vi "write asci file.vi"(5 "Temp in":T1={"Vibr Chn Name"=[], "Analysis Chn Number"=0, "Index Vibration Waveform"={"t0"=timestamp(0 s since 1904-01-01), "dt"=1.0, "Y"=[]}, "Report Infomation"={"Test Name"="", "Tester"="", "Tempre Chart"=refnum, "Apli-Fre"=refnum, "Phase-Fre"=refnum, "Raw Data"=refnum}, "Vibr Apli - Fre"=[], "Vibr Phase - Fre"=[], "Error"={"status"=FALSE, "code"=0, "source"=""}, "Read Chan Name"="", "Test Info"={"Test Name"="", "Tester"=""}, "test data"=[{"t0"=timestamp(0 s since 1904-01-01), "dt"=1.0, "Y"=[]}, {"t0"=timestamp(0 s since 1904-01-01), "dt"=1.0, "Y"=[]}, {"t0"=timestamp(0 s since 1904-01-01), "dt"=1.0, "Y"=[]}, {"t0"=timestamp(0 s since 1904-01-01), "dt"=0.001, "Y"=[]}], "测试头文件"={"ch"=[], "测试环境"=""}, "CAl VAlUE"={"max_t"=[], "max_V"=[], "start_t"=[], "start_V"=[], "distance"=[], "unit"=""}}, 6 "unit":string[](array[string]), 7 "chanel name":string[](array[string]), 8 "error in (no error)":errorcluster, 9 "data":waveform(dbl)[](array[waveform]), 10 "格式":string, 11 "file (use dialog)":path) -> (0 "error out":errorcluster)   [LabVIEW 2011]
uses:
  Ctrls/ana data.ctl
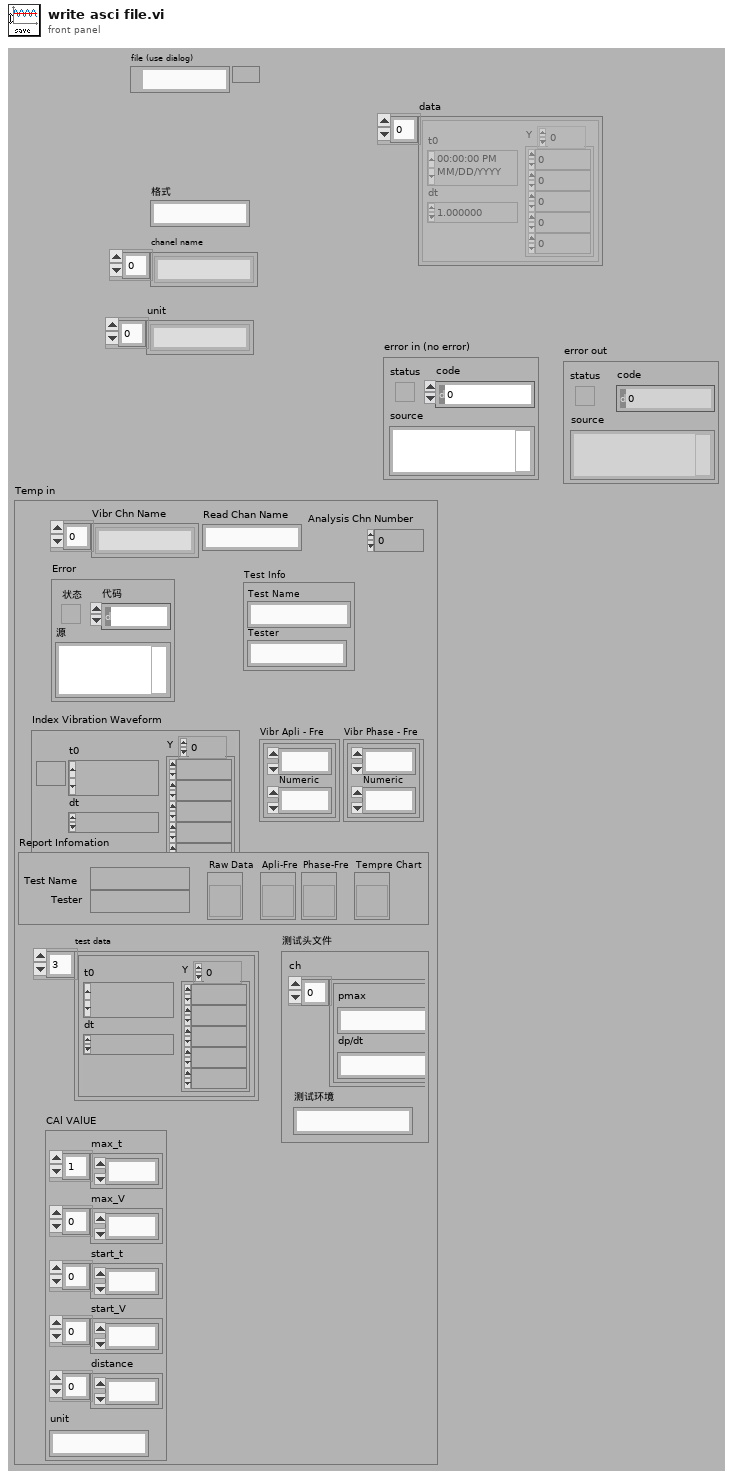
[diagram p1: front panel]
types:
  T1 = typedef "ana data.ctl" = cluster{"Vibr Chn Name":string[], "Analysis Chn Number":i32, "Index Vibration Waveform":waveform(dbl), "Report Infomation":cluster{"Test Name":string, "Tester":string, "Tempre Chart":refnum<vi>, "Apli-Fre":refnum<vi>, "Phase-Fre":refnum<vi>, "Raw Data":refnum<vi>}, "Vibr Apli - Fre":cluster{dbl, "Numeric":dbl}[], "Vibr Phase - Fre":cluster{dbl, "Numeric":dbl}[], "Error":errorcluster, "Read Chan Name":string, "Test Info":cluster{"Test Name":string, "Tester":string}, "test data":waveform(dbl)[], "测试头文件":cluster{"ch":cluster{"pmax":string, "dp/dt":string}[], "测试环境":string}, "CAl VAlUE":cluster{"max_t":dbl[], "max_V":dbl[], "start_t":dbl[], "start_V":dbl[], "distance":dbl[], "unit":string}}
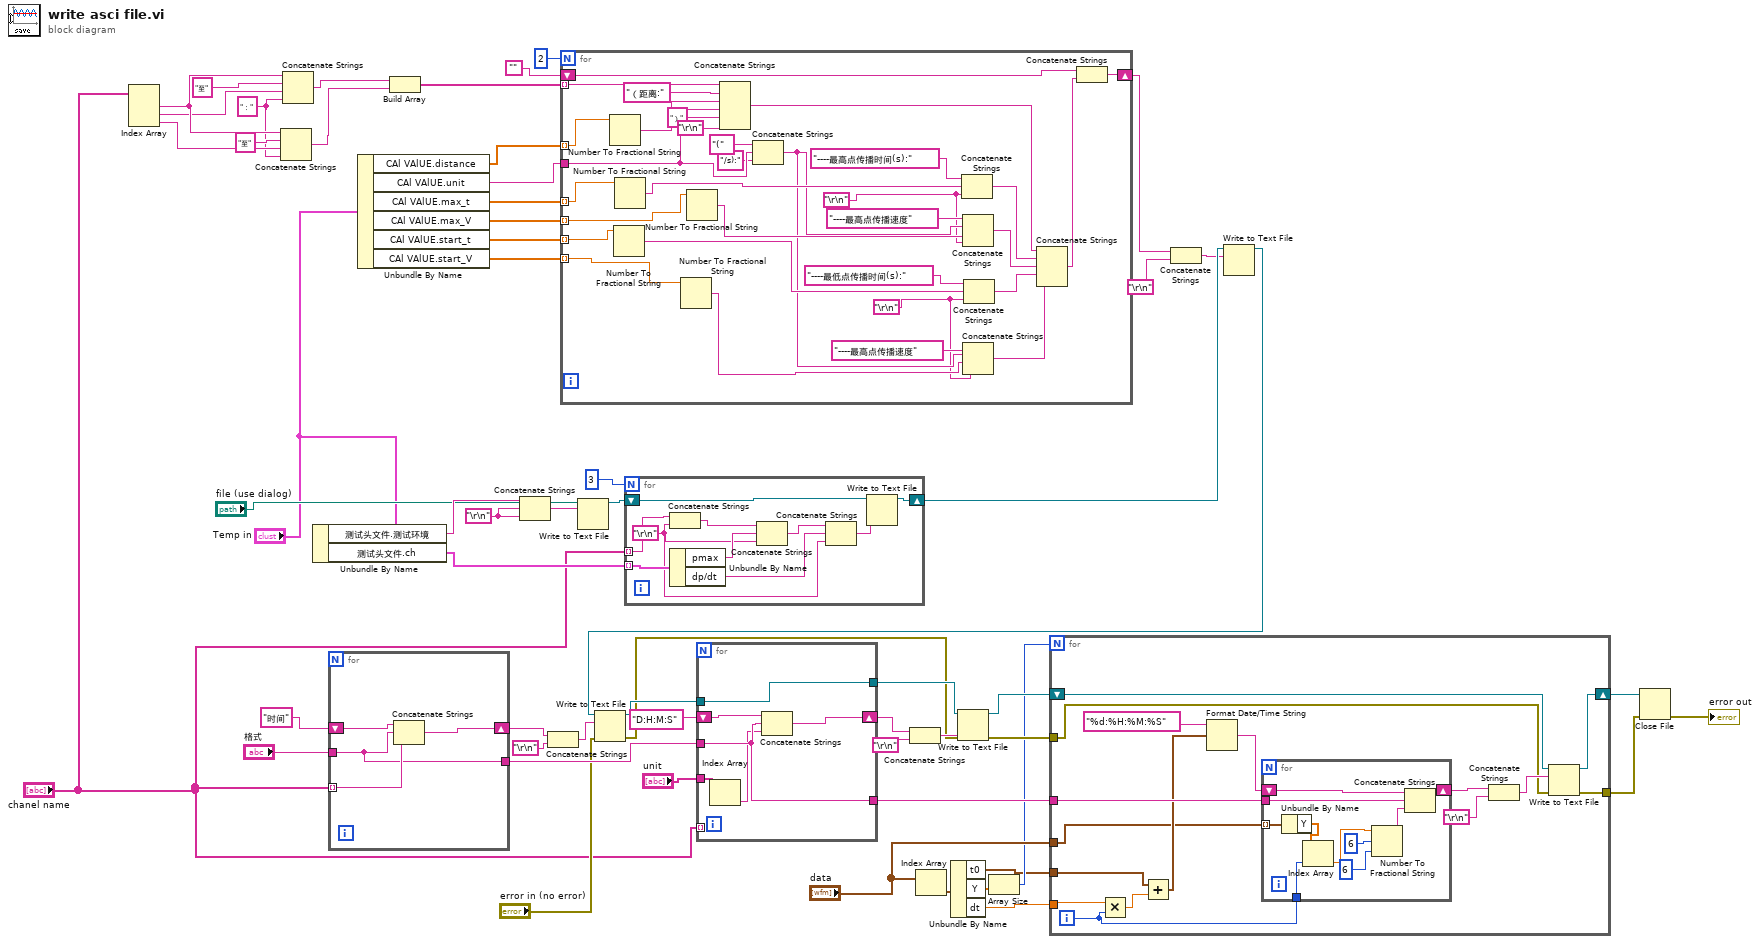
[diagram p0: block diagram]
diagram:
  w10 = "：" ("字符串")
  w25 = "\r\n"
  n1 = Index Array(array="chanel name") -> (element #1=w14:string, element #2=w12:string, element #3=w11:string)  [unwired: 3 in]
  n2 = Concatenate Strings(w14, "至" ("字符串"), w11, w10) -> (w8:string)
  n3 = Concatenate Strings(w14, "至" ("字符串"), w12, w10) -> (w9:string)
  n4 = Unbundle By Name("Temp in") -> ("测试头文件.测试环境"=w31:string, "测试头文件.ch"=w29:cluster{"pmax":string, "dp/dt":string}[])
  n5 = for {
    tunnel: "chanel name" -> [w60] mode=indexing
    shift-right: [w61] -> w55
    shift-left: "时间" -> [w62]
    tunnel: "格式" -> [w59]
    tunnel: [w59] -> w52
    n6 = Concatenate Strings(w62, w59, w60) -> (w61:string)
  }
  n7 = Unbundle By Name("Temp in") -> ("CAl VAlUE.distance"=w22:dbl[], "CAl VAlUE.unit"=w21:string, "CAl VAlUE.max_t"=w20:dbl[], "CAl VAlUE.max_V"=w19:dbl[], "CAl VAlUE.start_t"=w18:dbl[], "CAl VAlUE.start_V"=w17:dbl[])
  n8 = Build Array(w9, w8) -> (w7:string[])
  n9 = Concatenate Strings(w31, w25, w25) -> (w26:string)
  n10 = Concatenate Strings(w55, "\r\n") -> (w56:string)
  n11 = for {
    N: 2 -> [_]
    tunnel: w22 -> [w93] mode=indexing
    tunnel: w21 -> [w87]
    tunnel: w20 -> [w91] mode=indexing
    tunnel: w19 -> [w90] mode=indexing
    tunnel: w18 -> [w89] mode=indexing
    tunnel: w17 -> [w88] mode=indexing
    tunnel: w7 -> [w94] mode=indexing
    shift-right: [w68] -> w5
    shift-left: "" -> [w67]
    w74 = "\r\n"
    w75 = "\r\n"
    n12 = Number To Fractional String(number=w93) -> (F-format string=w92:string)  [unwired: 3 out]
    n13 = Number To Fractional String(number=w89) -> (F-format string=w79:string)  [unwired: 3 out]
    n14 = Number To Fractional String(number=w91) -> (F-format string=w84:string)  [unwired: 3 out]
    n15 = Number To Fractional String(number=w88) -> (F-format string=w76:string)  [unwired: 3 out]
    n16 = Number To Fractional String(number=w90) -> (F-format string=w81:string)  [unwired: 3 out]
    n17 = Concatenate Strings(w94, "（距离:" ("字符串"), w92, w87, "）" ("字符串"), "\r\n") -> (w69:string)
    n18 = Concatenate Strings("(" ("字符串"), w87, "/s):" ("字符串")) -> (w77:string)
    n19 = Concatenate Strings("----最高点传播时间(s):" ("字符串"), w84, w75) -> (w73:string)
    n20 = Concatenate Strings("----最高点传播速度" ("字符串"), w77, w81, w75) -> (w72:string)
    n21 = Concatenate Strings("----最高点传播速度" ("字符串"), w77, w76, w74) -> (w70:string)
    n22 = Concatenate Strings("----最低点传播时间(s):" ("字符串"), w79, w74) -> (w71:string)
    n23 = Concatenate Strings(w69, w73, w72, w71, w70) -> (w66:string)
    n24 = Concatenate Strings(w67, w66) -> (w68:string)
  }
  n25 = Write to Text File(file (use dialog)="file (use dialog)", text=w26) -> (refnum out=w30:refnum<file>)  [unwired: 1 in, 3 out]
  n26 = for {
    N: 3 -> [_]
    shift-right: [w102] -> w4
    shift-left: w30 -> [w95]
    tunnel: w29 -> [w103] mode=indexing
    tunnel: "chanel name" -> [w104] mode=indexing
    w99 = "\r\n"
    n27 = Concatenate Strings(w104, w99) -> (w97:string)
    n28 = Unbundle By Name(w103) -> ("pmax"=w101:string, "dp/dt"=w100:string)
    n29 = Concatenate Strings(w97, w101, w99) -> (w96:string)
    n30 = Concatenate Strings(w96, w100, w99) -> (w98:string)
    n31 = Write to Text File(file (use dialog)=w95, text=w98) -> (refnum out=w102:refnum<file>)  [unwired: 1 in, 3 out]
  }
  n32 = Index Array(array="data") -> (element=w36:waveform(dbl))  [unwired: 1 in]
  n33 = Unbundle By Name(w36) -> ("t0"=w32:timestamp, "Y"=w35:dbl[], "dt"=w33:dbl)
  n34 = Array Size(array=w35) -> (size(s)=w34:i32)
  n35 = Concatenate Strings(w5, "\r\n") -> (w2:string)
  n36 = Write to Text File(file (use dialog)=w4, text=w2) -> (refnum out=w3:refnum<file>)  [unwired: 1 in, 3 out]
  n37 = Write to Text File(file (use dialog)=w3, text=w56, error in="error in (no error)") -> (refnum out=w46:refnum<file>, error out=w40:errorcluster)  [unwired: 2 out]
  n38 = for {
    tunnel: "unit" -> [w106]
    shift-right: [w109] -> w50
    shift-left: "D:H:M:S" -> [w110]
    tunnel: w52 -> [w107]
    tunnel: [w108] -> w47
    tunnel: w46 -> [w108]
    tunnel: [w107] -> w44
    tunnel: "chanel name" -> [_] mode=indexing
    n39 = Index Array(array=w106) -> (element=w105:string)  [unwired: 1 in]
    n40 = Concatenate Strings(w110, w107, w105) -> (w109:string)
  }
  n41 = Concatenate Strings(w50, "\r\n") -> (w48:string)
  n42 = Write to Text File(file (use dialog)=w47, text=w48, error in=w40) -> (refnum out=w45:refnum<file>, error out=w41:errorcluster)  [unwired: 2 out]
  n43 = for {
    N: w34 -> [_]
    shift-right: [w121] -> w43
    shift-left: w45 -> [w122]
    tunnel: w44 -> [w126]
    tunnel: [w118] -> w42
    tunnel: w41 -> [w117]
    tunnel: "data" -> [w112]
    tunnel: w33 -> [w116]
    tunnel: w32 -> [w114]
    i -> [w111]
    n44 = Multiply(x=w116, y=w111) -> (x*y=w115:dbl)
    n45 = Add(x=w114, y=w115) -> (x+y=w113:timestamp)
    n46 = Format Date/Time String(time format string (%c)="%d:%H:%M:%S", seconds (now)=w113) -> (date/time string=w120:string)  [unwired: 1 out]
    n47 = for {
      tunnel: w126 -> [w132]
      shift-right: [w131] -> w125
      shift-left: w120 -> [w136]
      tunnel: w112 -> [w130] mode=indexing
      tunnel: w111 -> [w128]
      n48 = Unbundle By Name(w130) -> ("Y"=w129:dbl[])
      n49 = Index Array(array=w129, index=w128) -> (element=w127:dbl)
      n50 = Number To Fractional String(number=w127, width (-)=i16 6, precision (6)=i16 6) -> (F-format string=w133:string)  [unwired: 1 out]
      n51 = Concatenate Strings(w136, w132, w133) -> (w131:string)
    }
    n52 = Concatenate Strings(w125, "\r\n") -> (w123:string)
    n53 = Write to Text File(file (use dialog)=w122, text=w123, error in=w117) -> (refnum out=w121:refnum<file>, error out=w118:errorcluster)  [unwired: 2 out]
  }
  n54 = Close File(refnum=w43, error in=w42) -> (error out=→"error out":errorcluster)  [unwired: 1 out]
